vi "PAQ_Table_read_n_samples_from_end.vi"(8 "error in (no error)":errorcluster, 9 "Sub Path":path, 10 "Required samples":i32, 11 "Table Filename":string) -> (0 "error out":errorcluster, 1 "TAGs":string[](array[string]), 2 "Fetched samples":i32, 3 "value":T1)   [LabVIEW 2020, in "Sgraph_lib_V1.lvlib" / "DBAL-BIN.lvclass"]
uses:
  DBAL-BIN.lvclass
  controls/BIN/BINdata.ctl
  Common/controls/Global-test.vi
  Builds/Sgraph_lib_V1.lvlib
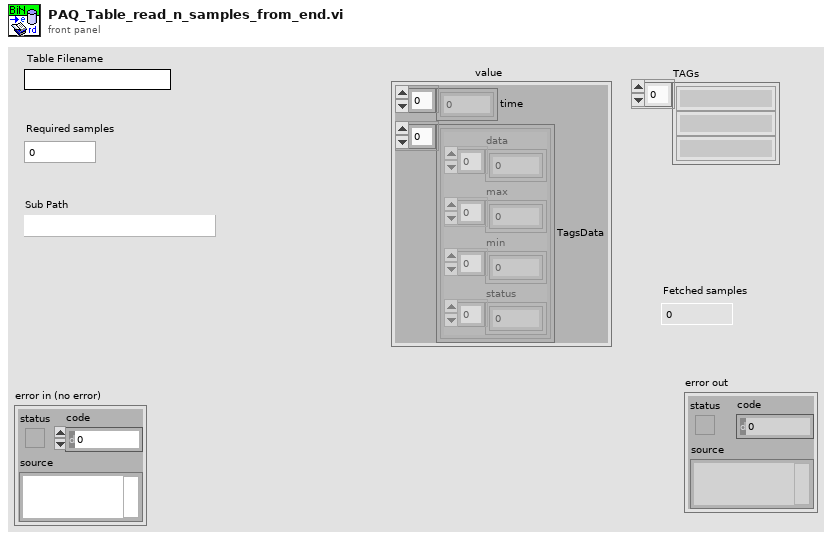
[diagram p1: front panel]
types:
  T1 = typedef "Sgraph_lib_V1.lvlib/DBAL-BIN.lvclass/BINdata.ctl" = cluster{"time":dbl[], "TagsData":cluster{"data":dbl[], "max":dbl[], "min":dbl[], "status":u32[]}[]}
  T2 = cluster{"data":dbl[], "max":dbl[], "min":dbl[], "status":u32[]}[]
  T3 = cluster{"data":dbl[], "max":dbl[], "min":dbl[], "status":u32[]}
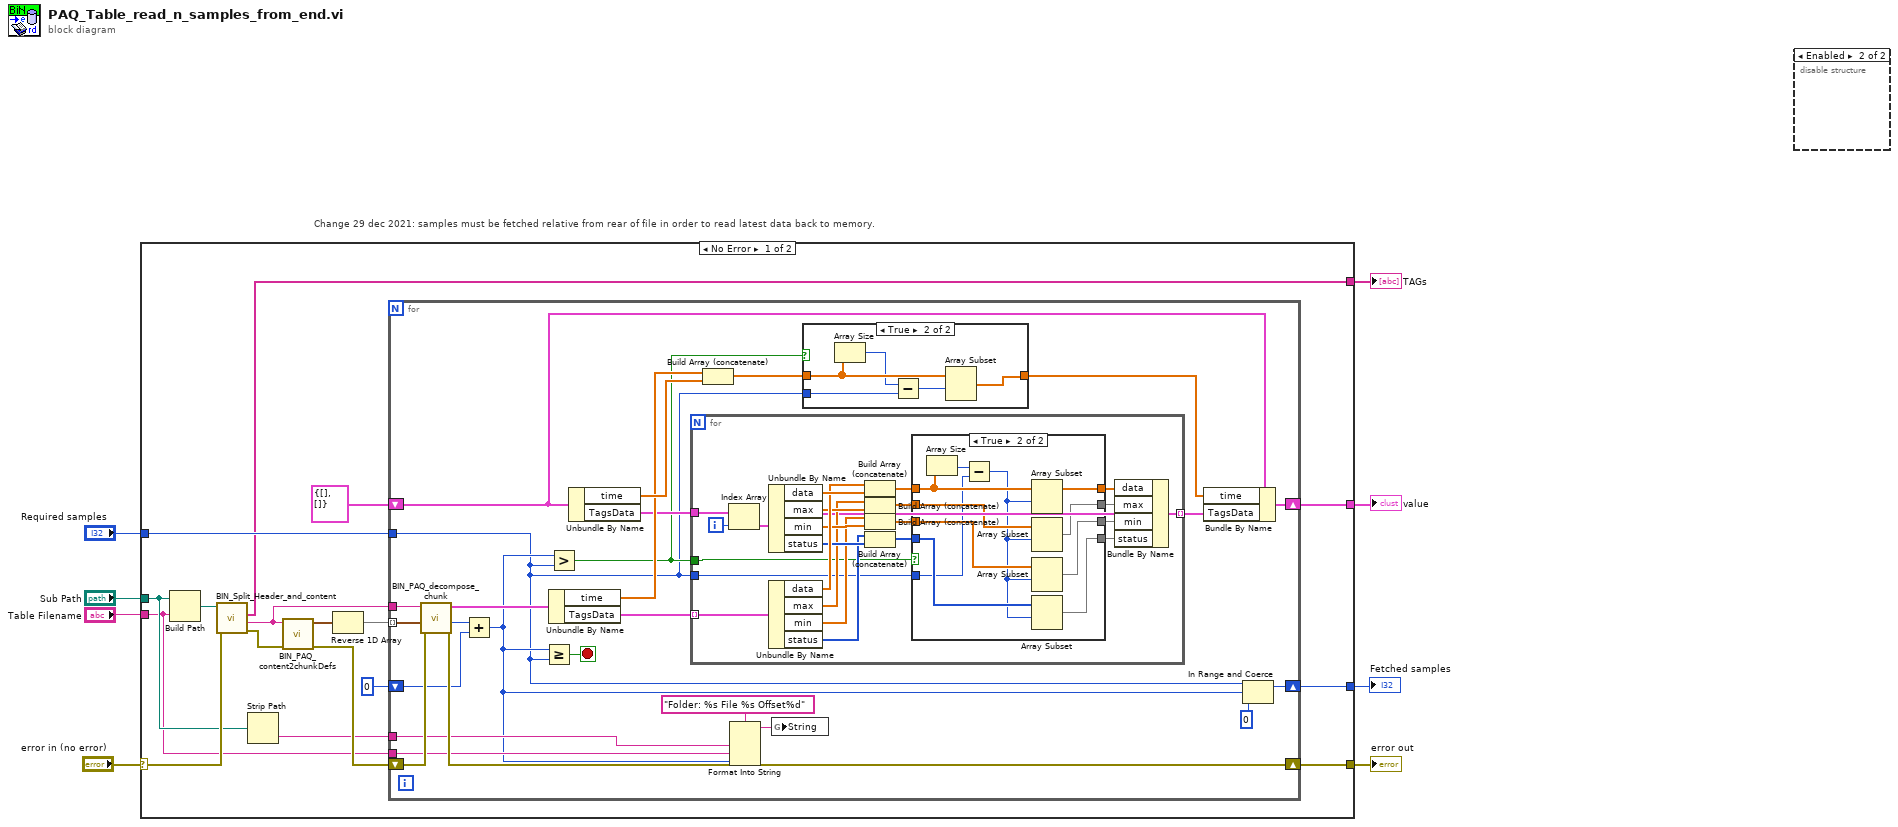
[diagram p0: block diagram]
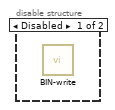
[diagram p2: hidden frame]
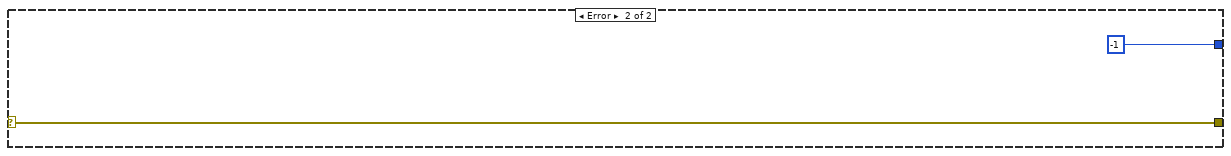
[diagram p5: hidden frame]
diagram:
  # "Change 29 dec 2021: samples must be fetched relative from rear of file in order to read latest data back to memory."
  n1 = case shown="No Error" "error in (no error)" {
    selector: "error in (no error)" -> [w24 w97]
    tunnel: [w20 w97] -> w7
    tunnel: "Sub Path" -> [w11 _]
    tunnel: "Table Filename" -> [w9 _]
    tunnel: "Required samples" -> [w18 _]
    tunnel: [w14 -1 ("Samples size")] -> w1
    tunnel: [w13 _] -> w3
    tunnel: [w12 _] -> w2
    frame No Error {
      n2 = Build Path(base path=w11, name or relative path=w9) -> (appended path=w25:path)
      n3 = call "BIN_Split_Header_and_content.vi"("error in"=w24, "Path in"=w25) -> ("error out"=w23:errorcluster, "Content"=w22:string, "TAGs"=w12:string[])  [unwired: 5 in, 2 out]
      n4 = Strip Path(path=w11) -> (name=w10:string)  [unwired: 1 out]
      n5 = call "BIN_PAQ_content2chunkDefs.vi"("error in (no error)"=w23, "Content"=w22) -> ("error out"=w21:errorcluster, "Data segments"=w19:cluster{"Offset":u32, "Size":u32}[])  [unwired: 8 in]
      n6 = Reverse 1D Array(array=w19) -> (reversed array=w17:cluster{"Offset":u32, "Size":u32}[])
      n7 = for {
        tunnel: w17 -> [w51] mode=indexing
        tunnel: w22 -> [w50]
        shift-right: [w48] -> w20
        shift-left: w21 -> [w49]
        tunnel: w18 -> [w26]
        shift-right: [w35] -> w14
        shift-left: 0 ("Samples size") -> [w36]
        shift-right: [w45] -> w13
        shift-left: T1 {"time"=[], "TagsData"=[]} ("PAQ_data") -> [w47]
        tunnel: w10 -> [w29]
        tunnel: w9 -> [w28]
        stop <- w39 stop-if-true
        n8 = call "BIN_PAQ_decompose_chunk.vi"("error in (no error)"=w49, "Offset"=w51, "Content"=w50) -> ("error out"=w48:errorcluster, "Samples size"=w37:i32, "PAQ_data"=w46:T1)  [unwired: 6 in]
        n9 = Add(x=w37, y=w36) -> (x+y=w27:i32)
        n10 = Greater Or Equal?(x=w27, y=w26) -> (x >= y?=w39:bool)
        n11 = Greater?(x=w27, y=w26) -> (0:w34:bool)
        n12 = Unbundle By Name(w46) -> ("time"=w43:dbl[], "TagsData"=w42:T2)
        n13 = Unbundle By Name(w47) -> ("time"=w44:dbl[], "TagsData"=w41:T2)
        n14 = for {
          tunnel: w42 -> [w78] mode=indexing
          tunnel: w41 -> [w80]
          tunnel: [w68] -> w40 mode=indexing
          tunnel: w34 -> [w67]
          tunnel: w26 -> [w58]
          i -> [w79]
          n15 = Index Array(array=w80, index=w79) -> (element=w69:T3)
          n16 = Unbundle By Name(w69) -> ("data"=w77:dbl[], "max"=w75:dbl[], "min"=w74:dbl[], "status"=w73:u32[])
          n17 = Unbundle By Name(w78) -> ("data"=w76:dbl[], "max"=w70:dbl[], "min"=w71:dbl[], "status"=w72:u32[])
          n18 = Build Array (concatenate)(w76, w77) -> (w59:dbl[])
          n19 = Build Array (concatenate)(w70, w75) -> (w66:dbl[])
          n20 = Build Array (concatenate)(w71, w74) -> (w64:dbl[])
          n21 = Build Array (concatenate)(w72, w73) -> (w65:u32[])
          n22 = case shown="True" w67 {
            tunnel: w59 -> [w82 w88]
            tunnel: w66 -> [w83 w94]
            tunnel: w65 -> [w81 w90]
            tunnel: w64 -> [w84 w91]
            tunnel: [w84 w92] -> w63
            tunnel: [w83 w93] -> w62
            tunnel: [w82 w95] -> w61
            tunnel: [w81 w89] -> w60
            tunnel: w58 -> [_ w86]
            frame False {
            }
            frame True {
              n23 = Array Size(array=w88) -> (size(s)=w87:i32)
              n24 = Subtract(x=w87, y=w86) -> (x-y=w85:i32)
              n25 = Array Subset(array=w88, index=w85) -> (w95:dbl[])  [unwired: 1 in]
              n26 = Array Subset(array=w94, index=w85) -> (w93:dbl[])  [unwired: 1 in]
              n27 = Array Subset(array=w91, index=w85) -> (w92:dbl[])  [unwired: 1 in]
              n28 = Array Subset(array=w90, index=w85) -> (w89:u32[])  [unwired: 1 in]
            }
          }
          n29 = Bundle By Name(cluster=w69, "data"=w61, "max"=w62, "min"=w63, "status"=w60) -> (w68:T3)
        }
        n30 = Build Array (concatenate)(w43, w44) -> (w33:dbl[])
        n31 = Format Into String(format string="Folder: %s File %s Offset%d", w29, w28, w27) -> (resulting string=w31:string)  [unwired: 2 in, 1 out]
        n32 = global write "Global-test.vi" "String"(w31) -> ()
        n33 = case shown="True" w34 {
          tunnel: w33 -> [w52 w56]
          tunnel: [w52 w57] -> w32
          tunnel: w26 -> [_ w54]
          frame False {
          }
          frame True {
            n34 = Array Size(array=w56) -> (size(s)=w55:i32)
            n35 = Subtract(x=w55, y=w54) -> (x-y=w53:i32)
            n36 = Array Subset(array=w56, index=w53) -> (w57:dbl[])  [unwired: 1 in]
          }
        }
        n37 = Bundle By Name(cluster=w47, "time"=w32, "TagsData"=w40) -> (w45:T1)
        n38 = In Range and Coerce(upper limit=w26, x=w27, lower limit=0) -> (coerced(x)=w35:i32)  [unwired: 1 out]
      }
    }
    frame Error {
    }
  }
  "error out" <- w7
  "Fetched samples" <- w1
  "TAGs" <- w2
  "value" <- w3
  n39 = disable-structure shown="Enabled" {
    frame Disabled {
      n40 = call "BIN-write.vi"() -> ()  [unwired: 9 in, 3 out]
    }
    frame Enabled {
    }
  }
